vi "Unwrap Phase - Continuous.vi"(1 "Reset":bool, 2 "Input Signal":waveform(dbl)) -> (0 "Phase Unwrapped":waveform(dbl))   [LabVIEW 2020]
uses:
  <vilib>/Analysis/NI_AALPro.lvlib
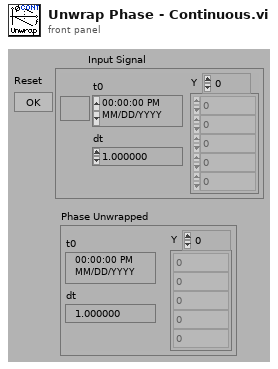
[diagram p1: front panel]
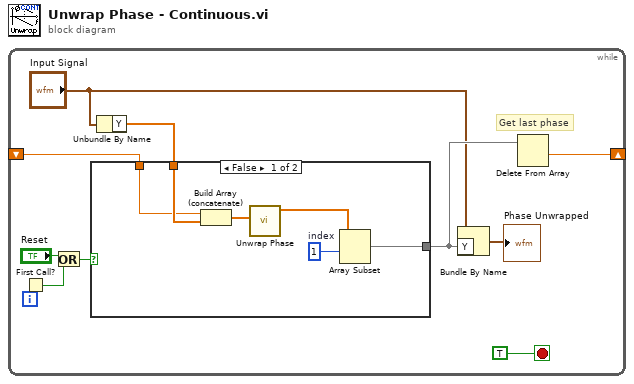
[diagram p0: block diagram]
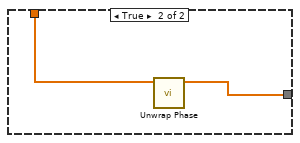
[diagram p2: hidden frame]
diagram:
  n1 = while {
    shift-right: [w9] -> _
    shift-left: _ -> [w8]
    stop <- TRUE stop-if-true
    # "Get last phase"
    n2 = First Call?() -> (First Call?: T/F=w6:bool)
    n3 = Or(x="Reset", y=w6) -> (x .or. y?=w5:bool)
    n4 = Unbundle By Name("Input Signal") -> ("Y"=w4:dbl[])
    n5 = case shown="False" w5 {
      tunnel: w4 -> [w16 w18]
      tunnel: [w15 w17] -> w2
      tunnel: w8 -> [w14 _]
      frame False {
        w11 = 1  # index
        n6 = Build Array (concatenate)(w14, w16) -> (w13:dbl[])
        n7 = call <vilib>:"Unwrap Phase.vi"("Phase"=w13) -> ("Unwrapped Phase"=w12:dbl[])  [unwired: 1 in, 9 out]
        n8 = Array Subset(array=w12, index=w11) -> (w15:dbl[])  [unwired: 1 in]
      }
      frame True {
        n9 = call <vilib>:"Unwrap Phase.vi"("Phase"=w18) -> ("Unwrapped Phase"=w17:dbl[])  [unwired: 1 in, 9 out]
      }
    }
    n10 = Bundle By Name(cluster="Input Signal", "Y"=w2) -> (→"Phase Unwrapped":waveform(dbl))
    n11 = Delete From Array(array=w2) -> (deleted portion=w9:dbl)  [unwired: 2 in, 1 out]
  }
